vi "fgt get valve position.vi"(8 "error in (no error)":errorcluster, 11 "valveIndex":u32) -> (0 "error out":errorcluster, 3 "position":i32)   [LabVIEW 2020, in "fgt_SDK.lvlib"]
doc: "Get the current position of the valve."
uses:
  fgt_SDK.lvlib
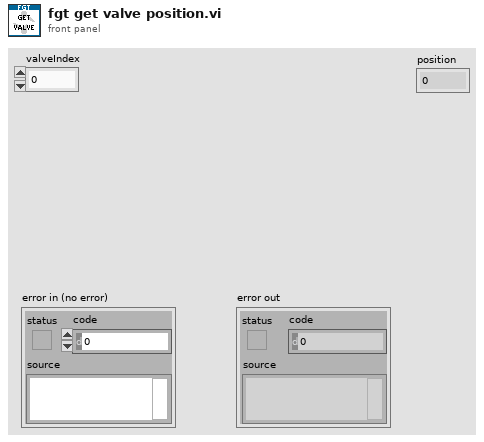
[diagram p1: front panel]
types:
  T1 = typedef "fgt_SDK.lvlib/fgt_STATUS_INFO.ctl" = cluster{"InstrType":T2, "instrSN":u16, "errorCode":u8, "infoCode":u8, "detail":string}
  T2 = typedef "fgt_SDK.lvlib/fgt_INSTRUMENT_TYPE.ctl" = enum32{"None", "MFCS", "MFCS_EZ", "FRP", "LineUP", "IPS"}
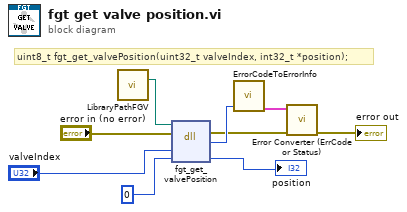
[diagram p0: block diagram]
diagram:
  # "uint8_t fgt_get_valvePosition(uint32_t valveIndex, int32_t *position);"
  n1 = call "LibraryPathFGV.vi"() -> ("Path Out"=w1:path)  [unwired: 14 in, 1 out]
  n2 = dll-call lib="C:/Workspace/fgt-SDK/LabVIEW/dlls/fgt_SDK_*.*" fn="fgt_get_valvePosition"(path in=w1, error in="error in (no error)", "valveIndex"="valveIndex", "position"=0) -> (error out=w5:errorcluster, "return type"=w7:u8, "position"=→"position":i32)  [unwired: 2 in, 1 out]
  n3 = call "ErrorCodeToErrorInfo.vi"("return type"=w7) -> ("StatusInfo"=w6:T1)  [unwired: 10 in]
  n4 = call "Error Converter (ErrCode or Status).vi"("error in (no error)"=w5, "StatusInfo"=w6) -> ("error out"=→"error out":errorcluster)  [unwired: 9 in]
